vi "macro_Pose3d_XYZ_RollPitchYaw_Deg.vi"   [LabVIEW 2019, in "Trajectory_Library.lvlib"]
uses:
  Trajectory_Library.lvlib
  Conv_Deg_Radians.vi
  VI/Quaternion_New.vi
  VI/Translation3d_Create.vi
  VI/Pose3d_New_Trans3dRot3d.vi
types:
  T1 = typedef "Trajectory_Library.lvlib/ROTATION3D.ctl" = cluster{"Q_quaternion":T2}
  T2 = typedef "Trajectory_Library.lvlib/QUATERNION.ctl" = cluster{"R":dbl, "V":dbl[]}
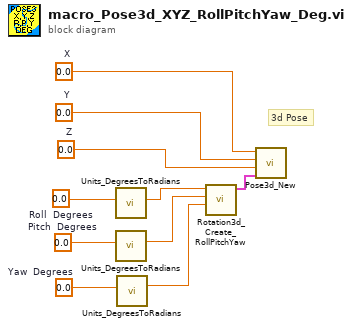
[diagram p0: block diagram]
diagram:
  w2 = 0.0  # X
  w3 = 0.0  # Y
  w4 = 0.0  # Z
  w10 = 0.0  # Roll  Degrees
  w9 = 0.0  # Pitch  Degrees
  w8 = 0.0  # Yaw  Degrees
  # "3d Pose"
  n1 = call "Units_DegreesToRadians.vi"("Degrees"=w10) -> ("Radians"=w7:dbl)  [unwired: 10 in]
  n2 = call "Units_DegreesToRadians.vi"("Degrees"=w9) -> ("Radians"=w6:dbl)  [unwired: 10 in]
  n3 = call "Units_DegreesToRadians.vi"("Degrees"=w8) -> ("Radians"=w5:dbl)  [unwired: 10 in]
  n4 = call "Rotation3d_Create_RollPitchYaw.vi"("Yaw"=w5, "Pitch"=w6, "Roll"=w7) -> ("Rotation3d"=w1:T1)  [unwired: 8 in]
  n5 = call "Pose3d_New.vi"("Rotation3d"=w1, "z"=w4, "Y"=w3, "X"=w2) -> ()  [unwired: 7 in, 1 out]
